vi "Initialise_Single_Puff.vi"() -> (5 "Plug in titles":string[](array[string]), 7 "Plug in values":string[](array[string]))   [LabVIEW 2012]
uses:
  Controls/Post_Process.ctl
  Globals/Meas_global.vi
panel:
  in  "Initial Purge (s)":u32=7
  out "Case Currently On":string="Set Acquisition interlock"
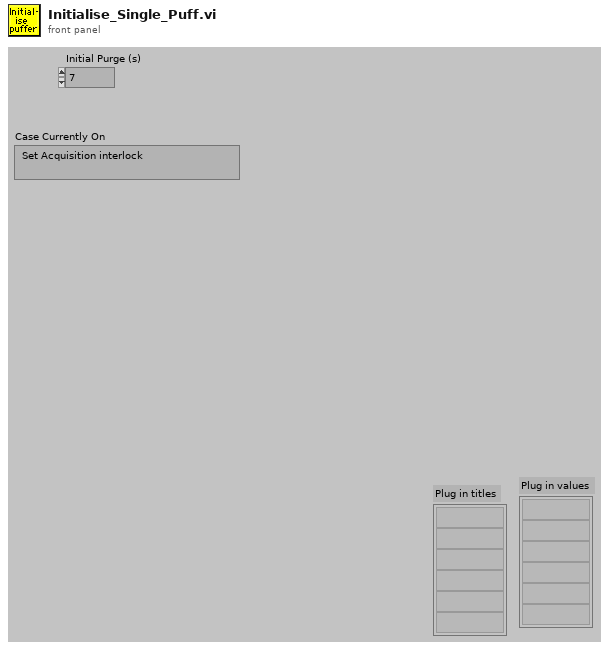
[diagram p1: front panel]
types:
  T1 = typedef "Post_Process.ctl" = enum16{"Take New Data", "Post Process Raw Data File"}
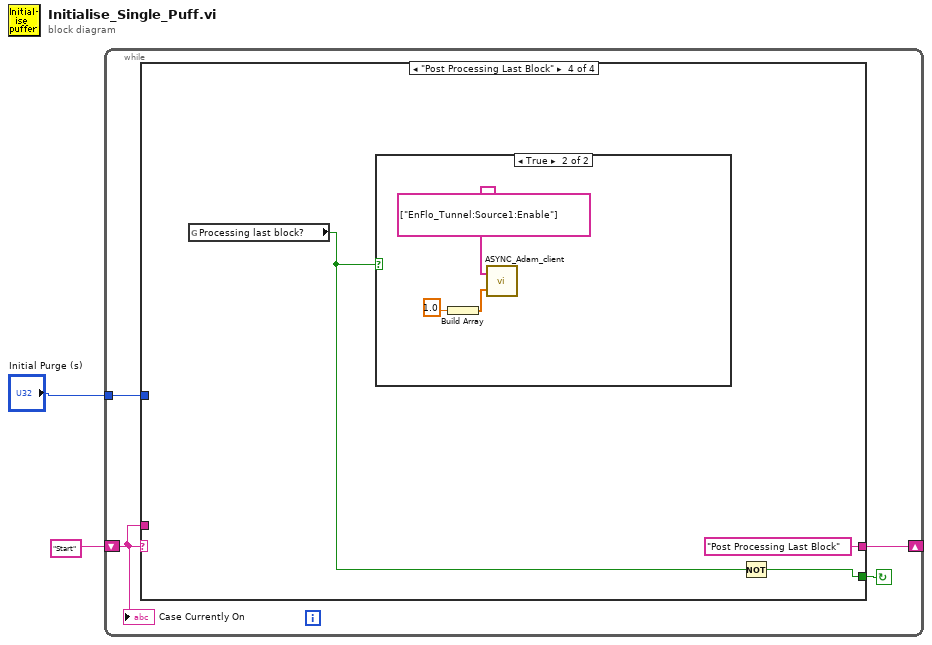
[diagram p0: block diagram]
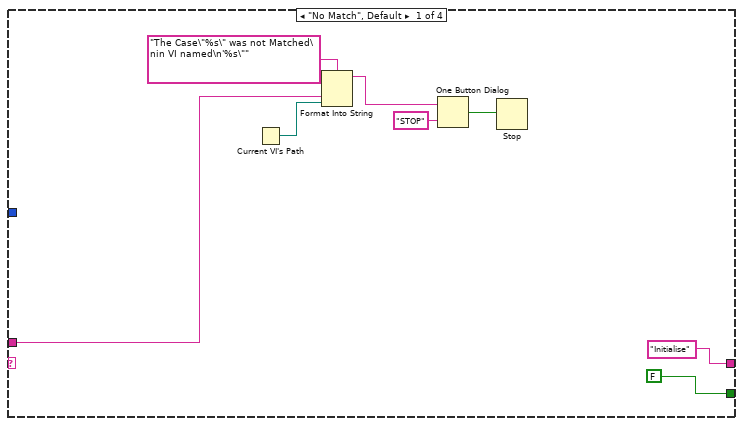
[diagram p2: hidden frame]
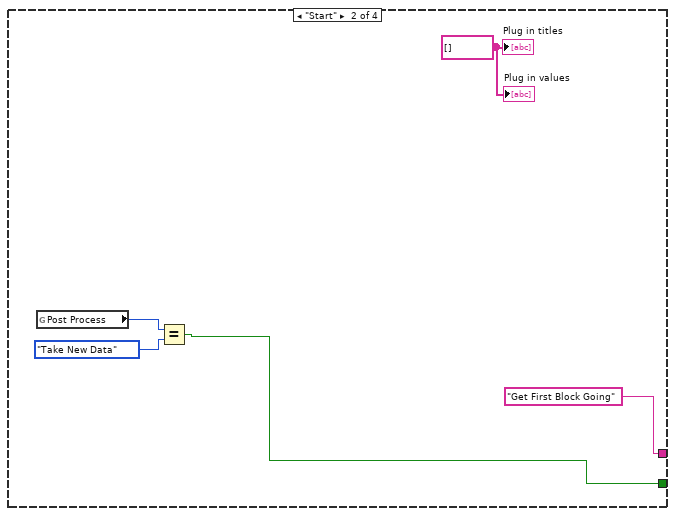
[diagram p3: hidden frame]
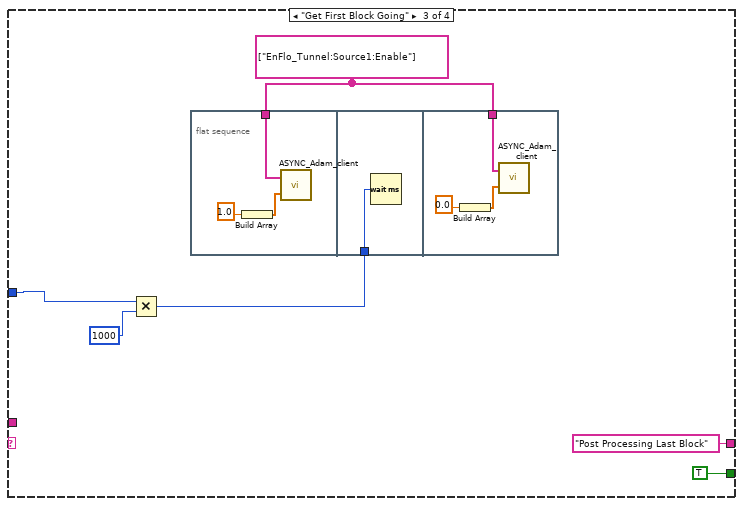
[diagram p4: hidden frame]
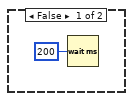
[diagram p5: hidden frame]
diagram:
  n1 = while {
    shift-left: "Start" -> [w4]
    shift-right: [w5] -> _
    tunnel: "Initial Purge (s)" -> [w3]
    stop <- w6 continue-if-true
    n2 = case shown="\"Post Processing Last Block\"" w4 {
      tunnel: [FALSE w15 TRUE ("Command Found") w33] -> w6
      tunnel: ["Initialise" "Get First Block Going" "Post Processing Last Block" "Post Processing Last Block"] -> w5
      tunnel: w4 -> [w9 _ _ _]
      tunnel: w3 -> [_ _ w23 _]
      frame "No Match", Default {
        n3 = Current VI's Path() -> (path=w8:path)
        n4 = Format Into String(format string="The Case\"%s\" was not Matched\nin VI named\n'%s\"" ("Format String"), w9, w8) -> (resulting string=w12:string)  [unwired: 2 in, 1 out]
        n5 = One Button Dialog(message=w12, button name ("OK")="STOP") -> (true=w10:bool)
        n6 = Stop(stop? (T)=w10) -> ()
      }
      frame "Start" {
        w16 = string[] [] ("Plug in titles")
        n7 = global read "Meas_global.vi" "Post Process"() -> (w17:T1)
        n8 = Equal?(x=w17, y=Post_Process."Take New Data" ("Post Process")) -> (x = y?=w15:bool)
        "Plug in values" <- w16
        "Plug in titles" <- w16
      }
      frame "Get First Block Going" {
        w20 = string[] ["EnFlo_Tunnel:Source1:Enable"] ("appended array")
        n9 = Multiply(x=w23, y=u32 1000) -> (x*y=w21:u32)
        n10 = flat-sequence {
          tunnel: w20 -> [w26]
          tunnel: w21 -> [w29]
          tunnel: w20 -> [w30]
          frame #0 {
            n11 = Build Array(1.0 ("New Value")) -> (w28:dbl[])
            n12 = call "ASYNC_Adam_client.vi"("Values"=w28, "Channel Names"=w26) -> ()  [unwired: 2 out]
          }
          frame #1 {
            n13 = Wait (ms)(milliseconds to wait=w29) -> ()  [unwired: 1 out]
          }
          frame #2 {
            n14 = Build Array(0.0 ("New Value")) -> (w31:dbl[])
            n15 = call "ASYNC_Adam_client.vi"("Values"=w31, "Channel Names"=w30) -> ()  [unwired: 2 out]
          }
        }
      }
      frame "Post Processing Last Block" {
        n16 = global read "Meas_global.vi" "Processing last block?"() -> (w34:bool)
        n17 = case shown="True" w34 {
          frame False {
            n18 = Wait (ms)(milliseconds to wait=u32 200) -> ()  [unwired: 1 out]
          }
          frame True {
            n19 = Build Array(1.0 ("New Value")) -> (w37:dbl[])
            n20 = call "ASYNC_Adam_client.vi"("Values"=w37, "Channel Names"=string[] ["EnFlo_Tunnel:Source1:Enable"] ("appended array")) -> ()  [unwired: 2 out]
          }
        }
        n21 = Not(x=w34) -> (.not. x?=w33:bool)
      }
    }
    "Case Currently On" <- w4
  }
